vi "Check Prime.vi"(11 "n":i64=1 min=0) -> (3 "prime?":bool)   [LabVIEW 2017, in "NI_AAL_MathFunc.lvlib"]
doc: "Returns TRUE if <b>n</b> is a prime number."
uses:
  <vilib>/gmath/NI_AAL_MathFunc.lvlib
panel:
  # "Check Prime?"
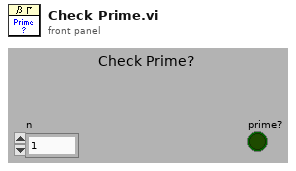
[diagram p1: front panel]
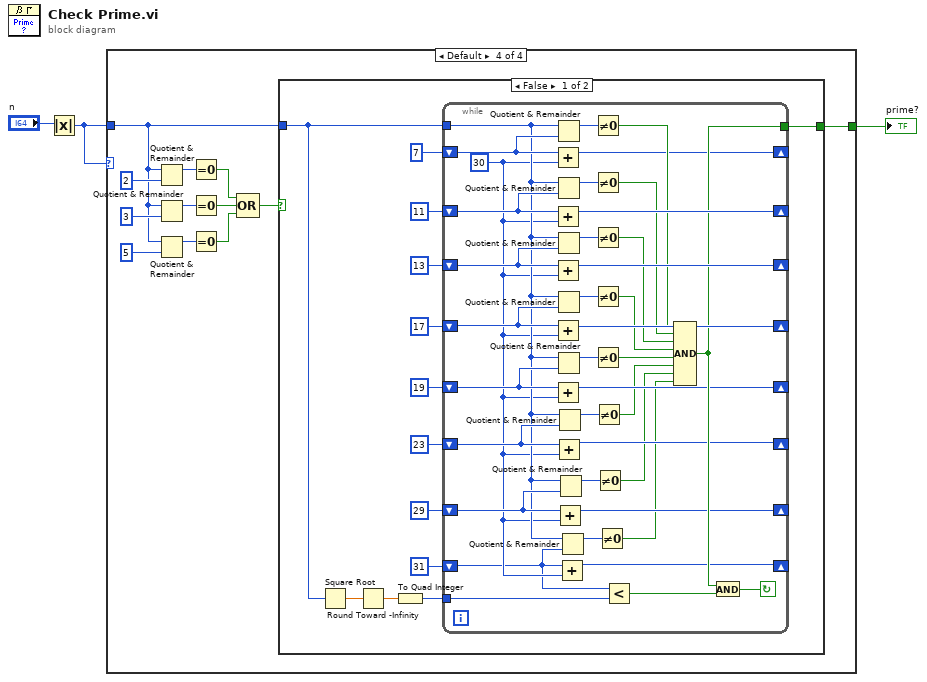
[diagram p0: block diagram]
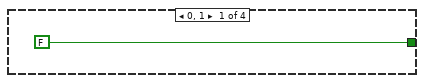
[diagram p2: hidden frame]
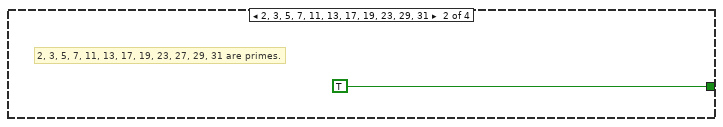
[diagram p3: hidden frame]
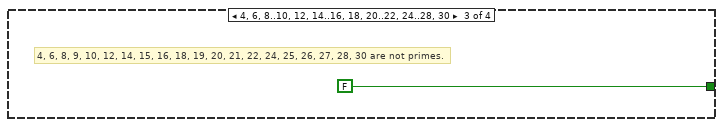
[diagram p4: hidden frame]
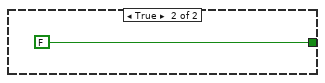
[diagram p5: hidden frame]
diagram:
  n1 = Absolute Value(x="n") -> (abs(x)=w2:i64)
  n2 = case shown="Default" w2 {
    tunnel: [FALSE TRUE FALSE w18] -> w1
    tunnel: w2 -> [_ _ _ w7]
    frame 0, 1 {
    }
    frame 2, 3, 5, 7, 11, 13, 17, 19, 23, 29, 31 {
      # "2, 3, 5, 7, 11, 13, 17, 19, 23, 27, 29, 31 are primes."
    }
    frame 4, 6, 8..10, 12, 14..16, 18, 20..22, 24..28, 30 {
      # "4, 6, 8, 9, 10, 12, 14, 15, 16, 18, 19, 20, 21, 22, 24, 25, 26, 27, 28, 30 are not primes."
    }
    frame Default {
      n3 = Quotient & Remainder(x=w7, y=i64 2) -> (x-y*floor(x/y)=w17:i64)  [unwired: 1 out]
      n4 = Quotient & Remainder(x=w7, y=i64 3) -> (x-y*floor(x/y)=w14:i64)  [unwired: 1 out]
      n5 = Quotient & Remainder(x=w7, y=i64 5) -> (x-y*floor(x/y)=w12:i64)  [unwired: 1 out]
      n6 = Equal To 0?(x=w17) -> (x = 0?=w11:bool)
      n7 = Equal To 0?(x=w14) -> (x = 0?=w10:bool)
      n8 = Equal To 0?(x=w12) -> (x = 0?=w9:bool)
      n9 = Compound Arithmetic op=OR(w11, w10, w9) -> (w8:bool)
      n10 = case shown="False" w8 {
        tunnel: [w30 FALSE] -> w18
        tunnel: w7 -> [w26 _]
        frame False {
          n11 = Square Root(x=w26) -> (sqrt(x)=w31:dbl)
          n12 = Round Toward -Infinity(1:w31) -> (0:w29:dbl)
          n13 = To Quad Integer(1:w29) -> (0:w28:i64)
          n14 = while {
            tunnel: w28 -> [w69]
            tunnel: w26 -> [w36]
            tunnel: [w52] -> w30
            shift-right: [w51] -> _
            shift-left: i64 7 -> [w67]
            shift-right: [w64] -> _
            shift-left: i64 11 -> [w66]
            shift-right: [w63] -> _
            shift-left: i64 13 -> [w61]
            shift-right: [w59] -> _
            shift-left: i64 17 -> [w50]
            shift-right: [w47] -> _
            shift-left: i64 19 -> [w48]
            shift-right: [w43] -> _
            shift-left: i64 23 -> [w44]
            shift-right: [w39] -> _
            shift-left: i64 29 -> [w40]
            shift-right: [w35] -> _
            shift-left: i64 31 -> [w32]
            stop <- w53 continue-if-true
            w34 = i64 30 ("x")
            n15 = Add(x=w67, y=w34) -> (x+y=w51:i64)
            n16 = Add(x=w66, y=w34) -> (x+y=w64:i64)
            n17 = Add(x=w61, y=w34) -> (x+y=w63:i64)
            n18 = Add(x=w50, y=w34) -> (x+y=w59:i64)
            n19 = Add(x=w48, y=w34) -> (x+y=w47:i64)
            n20 = Quotient & Remainder(x=w36, y=w67) -> (x-y*floor(x/y)=w68:i64)  [unwired: 1 out]
            n21 = Quotient & Remainder(x=w36, y=w66) -> (x-y*floor(x/y)=w65:i64)  [unwired: 1 out]
            n22 = Quotient & Remainder(x=w36, y=w61) -> (x-y*floor(x/y)=w62:i64)  [unwired: 1 out]
            n23 = Quotient & Remainder(x=w36, y=w50) -> (x-y*floor(x/y)=w60:i64)  [unwired: 1 out]
            n24 = Quotient & Remainder(x=w36, y=w48) -> (x-y*floor(x/y)=w49:i64)  [unwired: 1 out]
            n25 = Add(x=w44, y=w34) -> (x+y=w43:i64)
            n26 = Quotient & Remainder(x=w36, y=w44) -> (x-y*floor(x/y)=w45:i64)  [unwired: 1 out]
            n27 = Add(x=w40, y=w34) -> (x+y=w39:i64)
            n28 = Quotient & Remainder(x=w36, y=w40) -> (x-y*floor(x/y)=w41:i64)  [unwired: 1 out]
            n29 = Add(x=w32, y=w34) -> (x+y=w35:i64)
            n30 = Quotient & Remainder(x=w36, y=w32) -> (x-y*floor(x/y)=w37:i64)  [unwired: 1 out]
            n31 = Not Equal To 0?(x=w68) -> (x != 0?=w55:bool)
            n32 = Not Equal To 0?(x=w65) -> (x != 0?=w56:bool)
            n33 = Not Equal To 0?(x=w62) -> (x != 0?=w57:bool)
            n34 = Not Equal To 0?(x=w60) -> (x != 0?=w58:bool)
            n35 = Not Equal To 0?(x=w49) -> (x != 0?=w46:bool)
            n36 = Not Equal To 0?(x=w45) -> (x != 0?=w42:bool)
            n37 = Not Equal To 0?(x=w41) -> (x != 0?=w38:bool)
            n38 = Not Equal To 0?(x=w37) -> (x != 0?=w33:bool)
            n39 = Less?(x=w32, y=w69) -> (x < y?=w54:bool)
            n40 = Compound Arithmetic op=AND(w55, w56, w57, w58, w46, w42, w38, w33) -> (w52:bool)
            n41 = And(x=w52, y=w54) -> (x .and. y?=w53:bool)
          }
        }
        frame True {
        }
      }
    }
  }
  "prime?" <- w1
